vi "Refresh Database Cluster Comparison.vi"(8 "error in":errorcluster, 9 "CAN Cluster":T3, 10 "Refresh Listbox":T1={"Item Names"=[], "Item Symbols"=[enum."Port", enum."Incoming", enum."Outgoing", enum."Frame", enum."Signal", enum."Cluster"], "Change Flag"=[]}, 11 "Port Ref":T7 format="%.0x") -> (0 "error out":errorcluster, 2 "Refresh Listbox out":T1={"Item Names"=[], "Item Symbols"=[enum."Port", enum."Incoming", enum."Outgoing", enum."Frame", enum."Signal", enum."Cluster"], "Change Flag"=[]})   [LabVIEW 2020, in "Communication Bus Template System Explorer.lvlib" / "Implementation.lvlib"]
uses:
  <vilib>/NI VeriStand/Custom Device API/Custom Device Item Ref.ctl
  Types/Database.ctl
  Types/Frame.ctl
  Types/Signal.ctl
  Types/ECU.ctl
  Types/Refresh Listbox.ctl
  Types/Refresh Symbols.ctl
  Implementation.lvlib
  Scripting/Communication Bus Template Scripting.lvlib
  <vilib>/NI VeriStand/Custom Device API/Custom Device API.lvlib
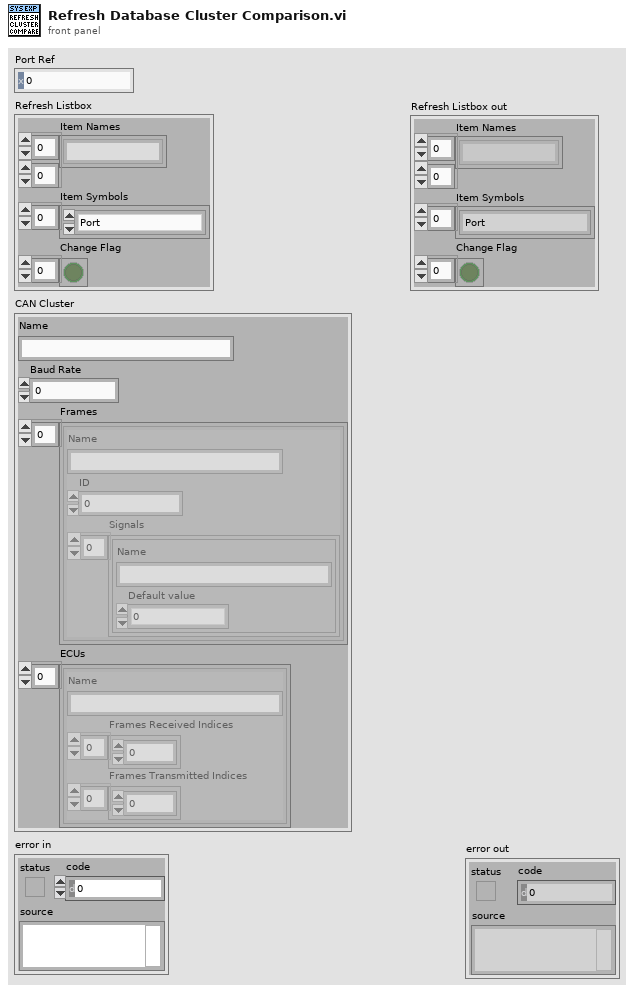
[diagram p1: front panel]
types:
  T1 = typedef "Communication Bus Template System Explorer.lvlib/Implementation.lvlib/Refresh Listbox.ctl" = cluster{"Item Names":string[][], "Item Symbols":T2[], "Change Flag":bool[]}
  T2 = typedef "Communication Bus Template System Explorer.lvlib/Implementation.lvlib/Refresh Symbols.ctl" = enum16{"Blank", "Port", "Incoming", "Outgoing", "Frame", "Signal", "Cluster", "Baud Rate"}
  T3 = typedef "Communication Bus Template System Explorer.lvlib/Implementation.lvlib/Database.ctl" = cluster{"Name":string, "Baud Rate":u64, "Frames":T4[], "ECUs":T6[]}
  T4 = typedef "Communication Bus Template System Explorer.lvlib/Implementation.lvlib/Frame.ctl" = cluster{"Name":string, "ID":u32, "Signals":T5[]}
  T5 = typedef "Communication Bus Template System Explorer.lvlib/Implementation.lvlib/Signal.ctl" = cluster{"Name":string, "Default value":dbl}
  T6 = typedef "Communication Bus Template System Explorer.lvlib/Implementation.lvlib/ECU.ctl" = cluster{"Name":string, "Frames Received Indices":u32[], "Frames Transmitted Indices":u32[]}
  T7 = typedef "Custom Device API.lvlib/Custom Device Item Ref.ctl" = u64
  T8 = typedef "Custom Device API.lvlib/Custom Device Channel.ctl" = cluster{"Type":T9, "Units":string, "Default Value":dbl, "Faultable":bool, "Scalable":bool}
  T9 = typedef "Custom Device API.lvlib/Custom Device Channel Type.ctl" = enum16{"Input", "Output"}
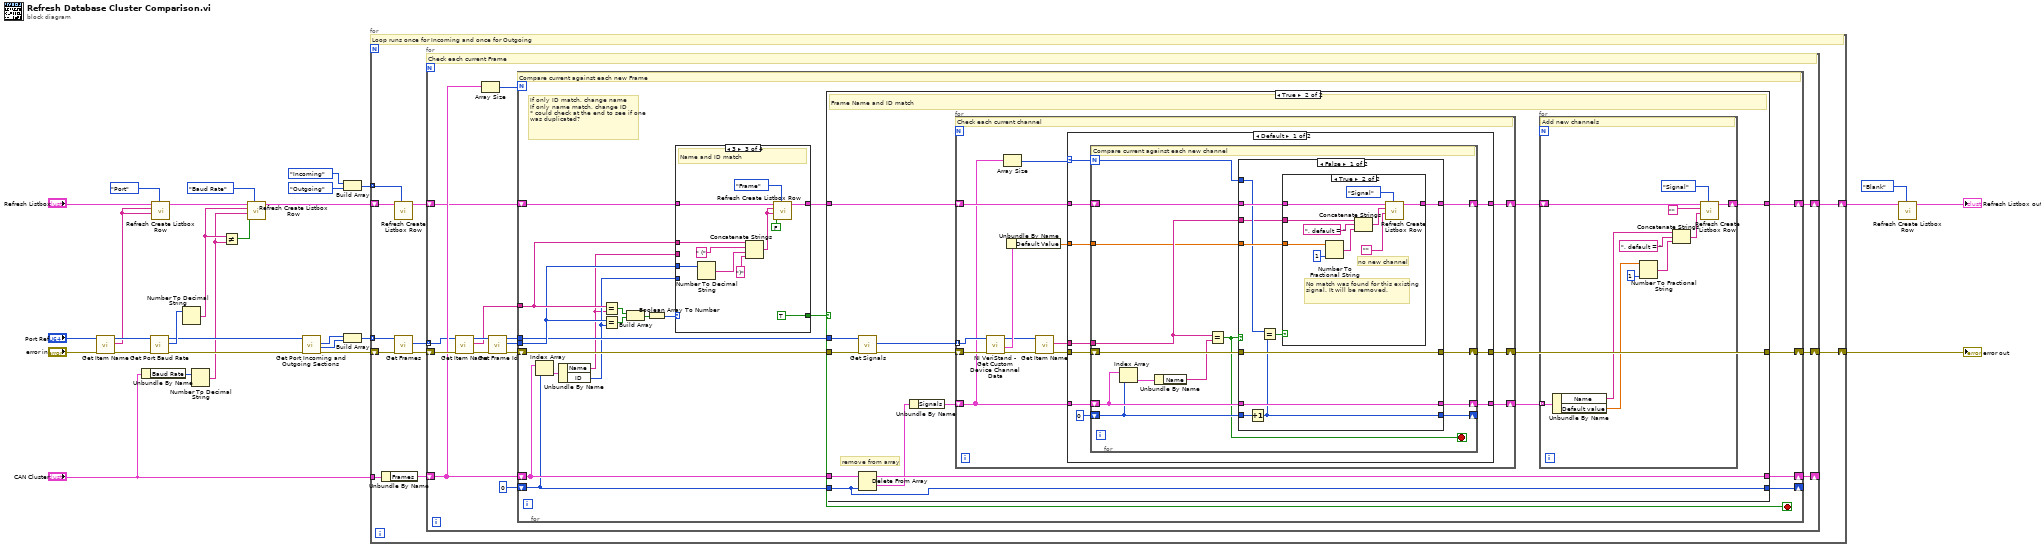
[diagram p0: block diagram]
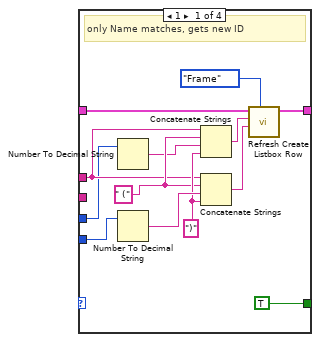
[diagram p2: hidden frame]
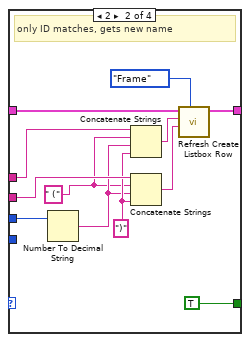
[diagram p3: hidden frame]
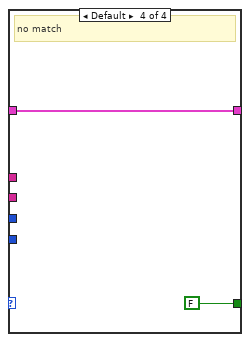
[diagram p4: hidden frame]
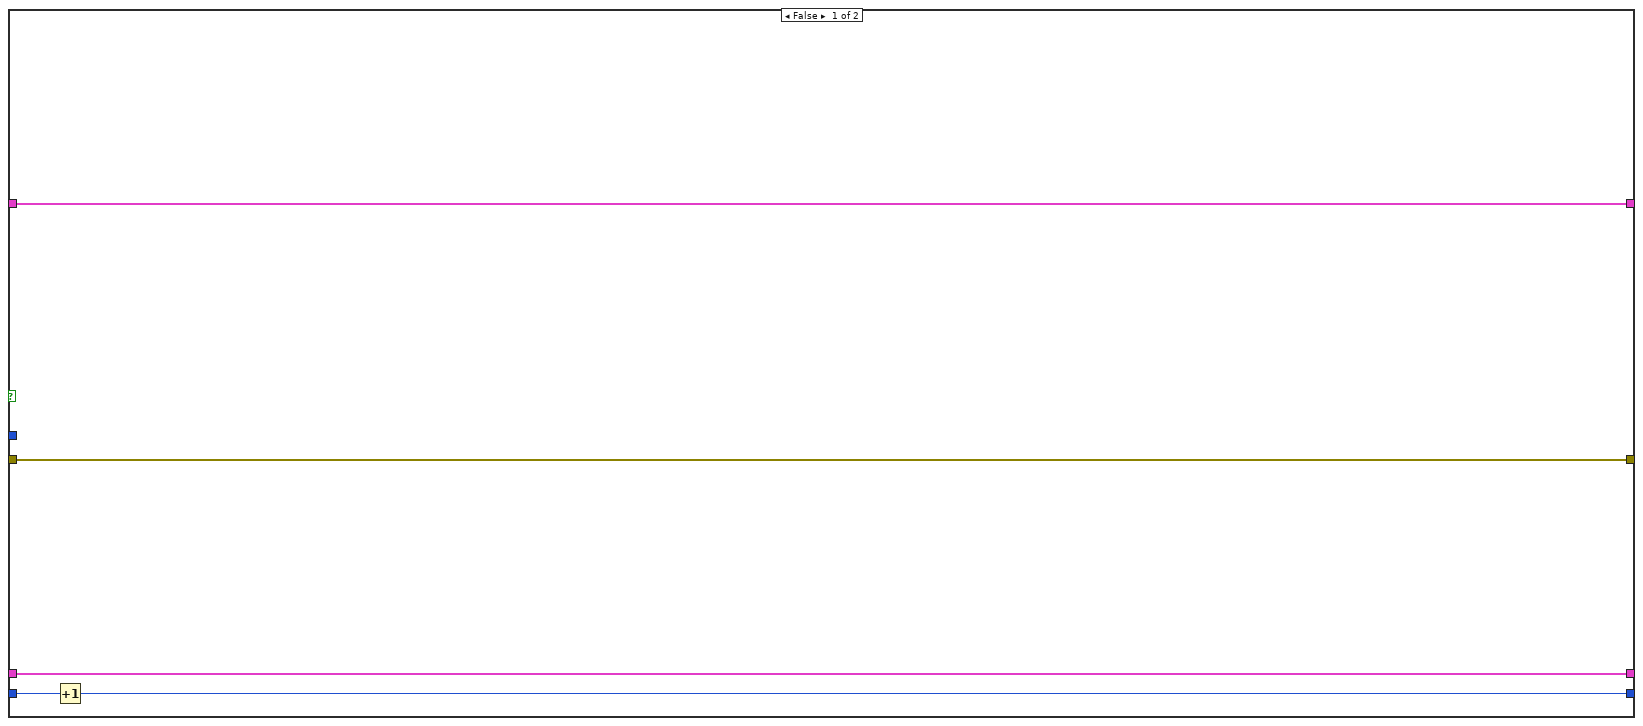
[diagram p5: hidden frame]
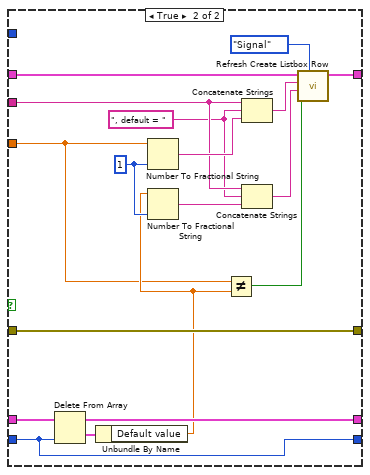
[diagram p7: hidden frame]
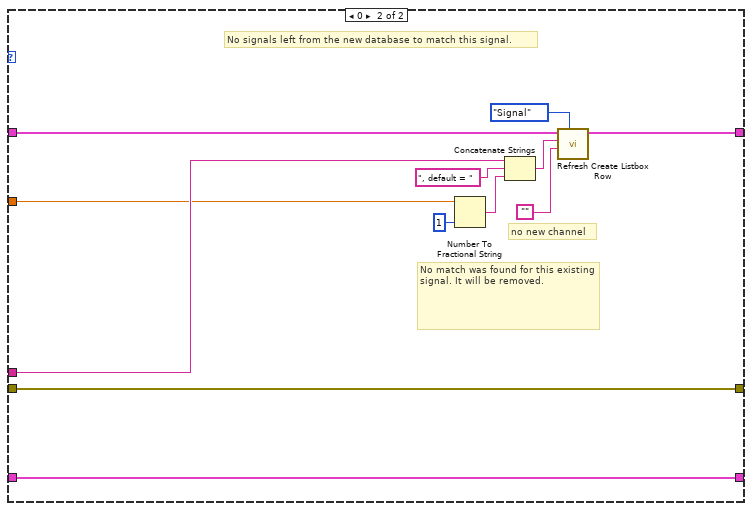
[diagram p8: hidden frame]
diagram:
  n1 = call "Get Item Name.vi"("error in"="error in", "Item Ref"="Port Ref") -> ("error out"=w12:errorcluster, "Name"=w4:string, "Item Ref out"=w11:T7)  [unwired: 7 in]
  n2 = Unbundle By Name("CAN Cluster") -> ("Baud Rate"=w29:u64)
  n3 = call "Get Port Baud Rate.vi"("error in"=w12, "Port Ref"=w11) -> ("error out"=w26:errorcluster, "Baud Rate"=w28:u32, "Port Ref out"=w27:T7)  [unwired: 7 in]
  n4 = call "Refresh Create Listbox Row.vi"("Refresh Symbol (Blank)"=Refresh_Symbols."Port" ("Refresh Symbols"), "New Item"=w4, "Old Item"=w4, "Refresh Listbox"="Refresh Listbox") -> ("Refresh Listbox out"=w8:T1)  [unwired: 7 in]
  n5 = Number To Decimal String(number=w28) -> (decimal integer string=w3:string)  [unwired: 1 in]
  n6 = Number To Decimal String(number=w29) -> (decimal integer string=w2:string)  [unwired: 1 in]
  n7 = Not Equal?(x=w3, y=w2) -> (x != y?=w1:bool)
  n8 = call "Refresh Create Listbox Row.vi"("Refresh Symbol (Blank)"=Refresh_Symbols."Baud Rate" ("Refresh Symbols"), "Change? (T)"=w1, "New Item"=w2, "Old Item"=w3, "Refresh Listbox"=w8) -> ("Refresh Listbox out"=w24:T1)  [unwired: 6 in]
  n9 = call "Get Port Incoming and Outgoing Sections.vi"("error in"=w26, "Port Ref"=w27) -> ("error out"=w23:errorcluster, "Outgoing"=w21:T7, "Incoming"=w22:T7)  [unwired: 6 in, 1 out]
  n10 = Build Array(Refresh_Symbols."Incoming" ("Refresh Symbols"), Refresh_Symbols."Outgoing" ("Refresh Symbols")) -> (w17:T2[])
  n11 = Build Array(w22, w21) -> (w20:T7[])
  n12 = for {
    shift-right: [w31] -> w15
    shift-left: w23 -> [w40]
    shift-right: [w32] -> w6
    shift-left: w24 -> [w38]
    tunnel: w20 -> [w39] mode=indexing
    tunnel: w17 -> [w37] mode=indexing
    tunnel: "CAN Cluster" -> [w36]
    # "Loop runs once for Incoming and once for Outgoing"
    n13 = Unbundle By Name(w36) -> ("Frames"=w34:T4[])
    n14 = call "Refresh Create Listbox Row.vi"("Refresh Symbol (Blank)"=w37, "Refresh Listbox"=w38) -> ("Refresh Listbox out"=w33:T1)  [unwired: 9 in]
    n15 = call "Get Frames.vi"("error in"=w40, "Incoming/Outgoing in"=w39) -> ("error out"=w35:errorcluster, "Frames"=w30:T7[])  [unwired: 7 in, 1 out]
    n16 = for {
      shift-right: [w44] -> w31
      shift-left: w35 -> [w55]
      tunnel: w30 -> [w42] mode=indexing
      shift-right: [w43] -> _
      shift-left: w34 -> [w49]
      shift-right: [w45] -> w32
      shift-left: w33 -> [w48]
      # "Check each current Frame"
      n17 = call "Get Item Name.vi"("error in"=w55, "Item Ref"=w42) -> ("error out"=w54:errorcluster, "Name"=w50:string, "Item Ref out"=w53:T7)  [unwired: 7 in]
      n18 = Array Size(array=w49) -> (size(s)=w41:i32)
      n19 = call "Get Frame Id.vi"("error in"=w54, "Frame Ref"=w53) -> ("error out"=w52:errorcluster, "ID"=w51:u32, "Frame Ref out"=w47:T7)  [unwired: 7 in]
      n20 = for {
        N: w41 -> [_]
        shift-right: [w64] -> w44
        shift-left: w52 -> [w69]
        shift-right: [w70] -> w43
        shift-left: w49 -> [w71]
        tunnel: w51 -> [w72]
        tunnel: w50 -> [w73]
        shift-right: [w67] -> w45
        shift-left: w48 -> [w74]
        tunnel: w47 -> [w68]
        shift-right: [w65] -> _
        shift-left: 0 -> [w66]
        stop <- w59 stop-if-true
        # "If only ID match, change name\nIf only name match, change ID\n* could check at the end to see if one was duplicated?"
        # "Compare current against each new Frame"
        n21 = Index Array(array=w71, index=w66) -> (element=w75:T4)
        n22 = Unbundle By Name(w75) -> ("Name"=w57:string, "ID"=w58:u32)
        n23 = Equal?(x=w73, y=w57) -> (x = y?=w63:bool)
        n24 = Equal?(x=w72, y=w58) -> (x = y?=w62:bool)
        n25 = Build Array(w63, w62) -> (w61:bool[])
        n26 = Boolean Array To Number(Boolean array=w61) -> (number=w56:u32)
        n27 = case shown="3" w56 {
          tunnel: w74 -> [w88 w100 w111 w113]
          tunnel: w73 -> [w80 w91 w110 _]
          tunnel: w72 -> [w78 w96 w109 _]
          tunnel: [w85 w98 w104 w113] -> w60
          tunnel: [TRUE TRUE TRUE FALSE] -> w59
          tunnel: w58 -> [w83 _ _ _]
          tunnel: w57 -> [_ w95 _ _]
          frame 1 {
            w82 = ")" ("string")
            w81 = " ("
            # "only Name matches, gets new ID"
            n28 = Number To Decimal String(number=w78) -> (decimal integer string=w79:string)  [unwired: 1 in]
            n29 = Number To Decimal String(number=w83) -> (decimal integer string=w87:string)  [unwired: 1 in]
            n30 = Concatenate Strings(w80, w81, w79, w82) -> (w77:string)
            n31 = Concatenate Strings(w80, w81, w87, w82) -> (w76:string)
            n32 = call "Refresh Create Listbox Row.vi"("Refresh Symbol (Blank)"=Refresh_Symbols."Frame", "New Item"=w76, "Old Item"=w77, "Refresh Listbox"=w88) -> ("Refresh Listbox out"=w85:T1)  [unwired: 7 in]
          }
          frame 2 {
            w94 = ")" ("string")
            w92 = " ("
            # "only ID matches, gets new name"
            n33 = Number To Decimal String(number=w96) -> (decimal integer string=w93:string)  [unwired: 1 in]
            n34 = Concatenate Strings(w91, w92, w93, w94) -> (w90:string)
            n35 = Concatenate Strings(w95, w92, w93, w94) -> (w89:string)
            n36 = call "Refresh Create Listbox Row.vi"("Refresh Symbol (Blank)"=Refresh_Symbols."Frame", "New Item"=w89, "Old Item"=w90, "Refresh Listbox"=w100) -> ("Refresh Listbox out"=w98:T1)  [unwired: 7 in]
          }
          frame 3 {
            # "Name and ID match"
            n37 = Number To Decimal String(number=w109) -> (decimal integer string=w108:string)  [unwired: 1 in]
            n38 = Concatenate Strings(w110, " (", w108, ")" ("string")) -> (w102:string)
            n39 = call "Refresh Create Listbox Row.vi"("Refresh Symbol (Blank)"=Refresh_Symbols."Frame", "Change? (T)"=FALSE, "New Item"=w102, "Old Item"=w102, "Refresh Listbox"=w111) -> ("Refresh Listbox out"=w104:T1)  [unwired: 6 in]
          }
          frame Default {
            # "no match"
          }
        }
        n40 = case shown="True" w59 {
          tunnel: w60 -> [w117 w119]
          tunnel: w71 -> [w118 w132]
          tunnel: w66 -> [w116 w124]
          tunnel: [w118 w131] -> w70
          tunnel: w69 -> [w114 w130]
          tunnel: w68 -> [_ w129]
          tunnel: [w117 w121] -> w67
          tunnel: [w115 w124] -> w65
          tunnel: [w114 w123] -> w64
          frame False {
            n41 = Increment(x=w116) -> (x+1=w115:i32)
          }
          frame True {
            # "remove from array"
            # "Frame Name and ID match"
            n42 = call "Get Signals.vi"("error in"=w130, "Frame in"=w129) -> ("error out"=w128:errorcluster, "Signals"=w127:T7[])  [unwired: 7 in, 1 out]
            n43 = Delete From Array(array=w132, index=w124) -> (deleted portion=w126:T4, array with subset deleted=w131:T4[])  [unwired: 1 in]
            n44 = Unbundle By Name(w126) -> ("Signals"=w125:T5[])
            n45 = for {
              shift-right: [w147] -> w122
              shift-left: w119 -> [w150]
              tunnel: w127 -> [w156] mode=indexing
              shift-right: [w145] -> w120
              shift-left: w125 -> [w149]
              shift-right: [w146] -> w123
              shift-left: w128 -> [w157]
              # "Check each current channel"
              n46 = call <vilib>:"NI VeriStand - Get Custom Device Channel Data.vi"("error in (no error)"=w157, "Channel Ref in"=w156) -> ("error out"=w153:errorcluster, "Channel"=w155:T8, "Channel Ref out"=w154:T7)  [unwired: 4 in, 3 out]
              n47 = Array Size(array=w149) -> (size(s)=w144:i32)
              n48 = Unbundle By Name(w155) -> ("Default Value"=w148:dbl)
              n49 = call "Get Item Name.vi"("error in"=w153, "Item Ref"=w154) -> ("error out"=w152:errorcluster, "Name"=w151:string)  [unwired: 7 in, 1 out]
              n50 = case shown="Default" w144 {
                selector: w144 -> [w158 _]
                tunnel: w152 -> [w167 w232]
                tunnel: w151 -> [w166 w231]
                tunnel: w150 -> [w164 w230]
                tunnel: w149 -> [w163 w229]
                tunnel: w148 -> [w162 w228]
                tunnel: [w161 w227] -> w147
                tunnel: [w160 w232] -> w146
                tunnel: [w159 w229] -> w145
                frame Default {
                  n51 = for {
                    N: w158 -> [w168]
                    shift-right: [w174] -> w159
                    shift-left: w163 -> [w178]
                    shift-right: [w169] -> w160
                    shift-left: w167 -> [w181]
                    tunnel: w166 -> [w173]
                    shift-right: [w175] -> _
                    shift-left: 0 -> [w176]
                    shift-right: [w170] -> w161
                    shift-left: w164 -> [w177]
                    tunnel: w162 -> [w171]
                    stop <- w172 stop-if-true
                    # "Compare current against each new channel"
                    n52 = Index Array(array=w178, index=w176) -> (element=w180:T5)
                    n53 = Unbundle By Name(w180) -> ("Name"=w179:string)
                    n54 = Equal?(x=w173, y=w179) -> (x = y?=w172:bool)
                    n55 = case shown="False" w172 {
                      tunnel: w181 -> [w186 w209]
                      tunnel: w178 -> [w191 w220]
                      tunnel: w177 -> [w190 w219]
                      tunnel: w176 -> [w182 w217]
                      tunnel: [w183 w217] -> w175
                      tunnel: [w191 w216] -> w174
                      tunnel: w173 -> [w184 w213]
                      tunnel: w171 -> [w187 w204]
                      tunnel: [w189 w210] -> w170
                      tunnel: w168 -> [w185 _]
                      tunnel: [w186 w209] -> w169
                      frame False {
                        n56 = Increment(x=w182) -> (x+1=w183:i32)
                        n57 = Equal?(x=w185, y=w183) -> (x = y?=w188:bool)
                        n58 = case shown="True" w188 {
                          tunnel: w190 -> [w192 w202]
                          tunnel: [w192 w201] -> w189
                          tunnel: w184 -> [_ w197]
                          tunnel: w187 -> [_ w196]
                          frame False {
                          }
                          frame True {
                            # "No match was found for this existing signal. It will be removed."
                            # "no new channel"
                            n59 = Number To Fractional String(number=w196, precision (6)=i16 1) -> (F-format string=w200:string)  [unwired: 2 in]
                            n60 = Concatenate Strings(w197, ", default = ", w200) -> (w194:string)
                            n61 = call "Refresh Create Listbox Row.vi"("Refresh Symbol (Blank)"=Refresh_Symbols."Signal", "New Item"="", "Old Item"=w194, "Refresh Listbox"=w202) -> ("Refresh Listbox out"=w201:T1)  [unwired: 7 in]
                          }
                        }
                      }
                      frame True {
                        w208 = i16 1 ("precision (6)")
                        w212 = ", default = "
                        n62 = Delete From Array(array=w220, index=w217) -> (deleted portion=w214:T5, array with subset deleted=w216:T5[])  [unwired: 1 in]
                        n63 = Unbundle By Name(w214) -> ("Default value"=w205:dbl)
                        n64 = Number To Fractional String(number=w204, precision (6)=w208) -> (F-format string=w215:string)  [unwired: 2 in]
                        n65 = Number To Fractional String(number=w205, precision (6)=w208) -> (F-format string=w211:string)  [unwired: 2 in]
                        n66 = Not Equal?(x=w204, y=w205) -> (x != y?=w203:bool)
                        n67 = Concatenate Strings(w213, w212, w215) -> (w207:string)
                        n68 = Concatenate Strings(w213, w212, w211) -> (w206:string)
                        n69 = call "Refresh Create Listbox Row.vi"("Refresh Symbol (Blank)"=Refresh_Symbols."Signal", "Change? (T)"=w203, "New Item"=w206, "Old Item"=w207, "Refresh Listbox"=w219) -> ("Refresh Listbox out"=w210:T1)  [unwired: 6 in]
                      }
                    }
                  }
                }
                frame 0 {
                  # "No signals left from the new database to match this signal."
                  # "No match was found for this existing signal. It will be removed."
                  # "no new channel"
                  n70 = Number To Fractional String(number=w228, precision (6)=i16 1) -> (F-format string=w226:string)  [unwired: 2 in]
                  n71 = Concatenate Strings(w231, ", default = ", w226) -> (w222:string)
                  n72 = call "Refresh Create Listbox Row.vi"("Refresh Symbol (Blank)"=Refresh_Symbols."Signal", "New Item"="", "Old Item"=w222, "Refresh Listbox"=w230) -> ("Refresh Listbox out"=w227:T1)  [unwired: 7 in]
                }
              }
            }
            n73 = for {
              shift-right: [w140] -> w121
              shift-left: w122 -> [w141]
              tunnel: w120 -> [w143] mode=indexing
              # "Add new channels"
              n74 = Unbundle By Name(w143) -> ("Name"=w137:string, "Default value"=w136:dbl)
              n75 = Number To Fractional String(number=w136, precision (6)=i16 1) -> (F-format string=w139:string)  [unwired: 2 in]
              n76 = Concatenate Strings(w137, ", default = ", w139) -> (w134:string)
              n77 = call "Refresh Create Listbox Row.vi"("Refresh Symbol (Blank)"=Refresh_Symbols."Signal", "New Item"=w134, "Old Item"="", "Refresh Listbox"=w141) -> ("Refresh Listbox out"=w140:T1)  [unwired: 7 in]
            }
          }
        }
      }
    }
  }
  "error out" <- w15
  n78 = call "Refresh Create Listbox Row.vi"("Refresh Symbol (Blank)"=Refresh_Symbols."Blank", "Refresh Listbox"=w6) -> ("Refresh Listbox out"=→"Refresh Listbox out":T1)  [unwired: 9 in]
